vi "Task Loop.vi"(8 "error in (no error)":errorcluster, 11 "BasicEventLogger in":refnum<class "BasicEventLogger.lvclass">) -> (0 "error out":errorcluster)   [LabVIEW 2020, in "Volatus.lvlib" / "BasicEventLogger.lvclass"]
uses:
  BasicEventLogger.lvclass
  BasicEventLogger.lvclass/BasicEventLogger.ctl
  Event Level.ctl
  Volatus.lvlib
  Event.ctl
panel:
  out "Events":T1[](array[typedef]) {"Time Stamp" format="%<%Y/%m/%d %H:%M:%S%3u>T"}
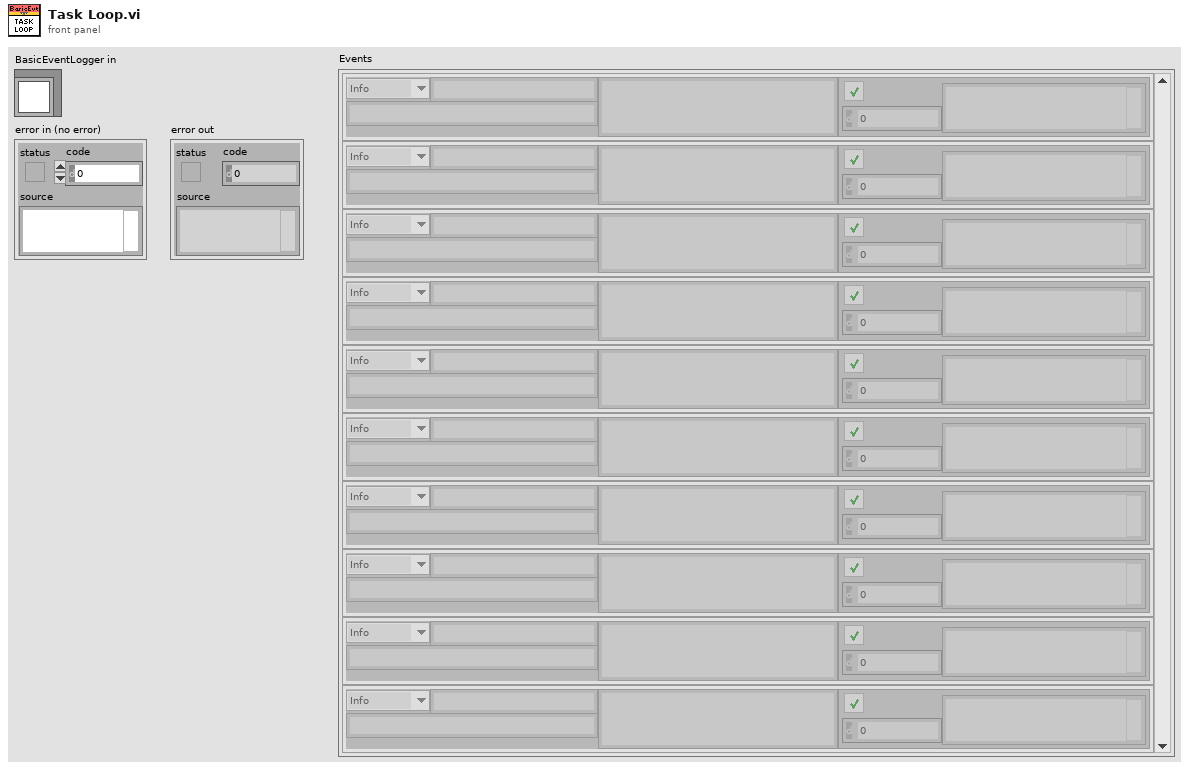
[diagram p1: front panel]
types:
  T1 = typedef "Volatus.lvlib/Event.ctl" = cluster{"Level":T2, "Context":string, "Message":string, "Error":errorcluster, "Time Stamp":timestamp}
  T2 = typedef "Volatus.lvlib/Event Level.ctl" = enum16{"Debug", "Info", "Warning", "Error"}
  T3 = enum32{"Invalid", "Standard", "Closed", "Hidden", "Minimized", "Maximized"}
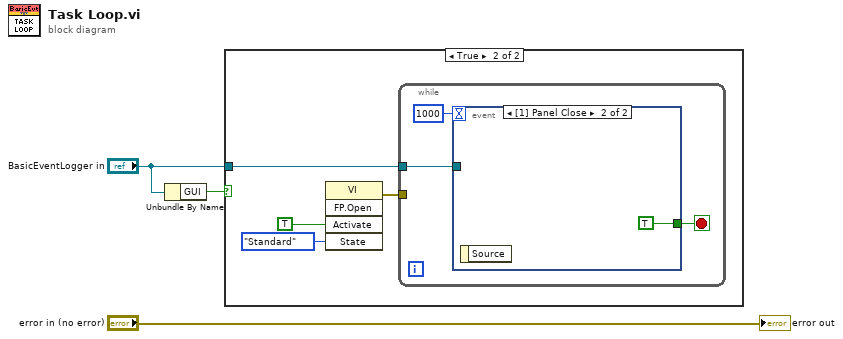
[diagram p0: block diagram]
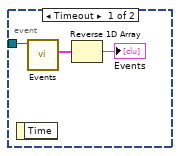
[diagram p3: hidden frame]
diagram:
  n1 = Unbundle By Name("BasicEventLogger in") -> ("GUI"=w2:bool)
  n2 = case shown="True" w2 {
    tunnel: "BasicEventLogger in" -> [_ w5]
    frame False {
    }
    frame True {
      n3 = invoke class="VI" method="FP.Open"("Activate"=TRUE ("Activate?"), "State"=T3."Standard") -> (error out=w4:errorcluster)  [unwired: 3 in, 4 out]
      n4 = while {
        tunnel: w5 -> [w10]
        tunnel: w4 -> [_]
        stop <- w8 stop-if-true
        n5 = event shown="[1] Panel Close" {
          selector: _ -> [_ _]
          dyn-events: _ -> [_ _]
          timeout: 1000 -> [_ _]
          tunnel: w10 -> [w13 _]
          tunnel: [_ TRUE] -> w8
          event Timeout {
            n6 = event-data() -> ()  [unwired: 1 in, 1 out]
            n7 = call-dynamic "Events.vi"("BasicEventLogger in"=w13) -> ("Events"=w12:T1[])  [unwired: 8 in, 2 out]
            n8 = Reverse 1D Array(array=w12) -> (reversed array=→"Events":T1[])
          }
          event Panel Close {
            n9 = event-data() -> ()  [unwired: 1 in, 1 out]
          }
        }
      }
    }
  }
  "error out" <- "error in (no error)"
